vi "Config CDMA Trigger.vi"(0 "VISA Resource Name":refnum<visa-resource-name>, 1 "Delay State (F: OFF)":bool, 2 "External Delay (0.002)":dbl=0.002, 5 "Trigger Source  (0: KEY)":u16(ring) items=["KEY", "External", "BUS"], 7 "Trigger Type  (0: Continuous)":i16(ring) items=["Continuous", "Single", "Gate", "Segment Advance"], 9 "Gate Active  (0: Low)":i16(ring) items=["Low", "High"], 11 "error in (no error)":errorcluster {"code" format="%.0x"}, 12 "External Polarity  (1: Negative)":i16(ring)=1 items=["Positive", "Negative"]) -> (4 "VISA Resource Name Out":refnum<visa-resource-name>, 15 "error out":errorcluster {"code" format="%.0x"})   [LabVIEW 2014, in "Agilent ESG Series.lvlib"]
doc: "This VI configures CDMA trigger parameters.\n\nNotes:\n(1) This VI is supported for Agilent E44xxB with options UND and UN5 or E4438C with option 401 only."
uses:
  Agilent ESG Series.lvlib
panel:
  # "ON"
  # "OFF"
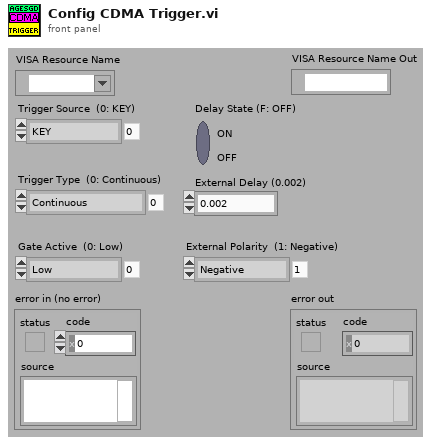
[diagram p1: front panel]
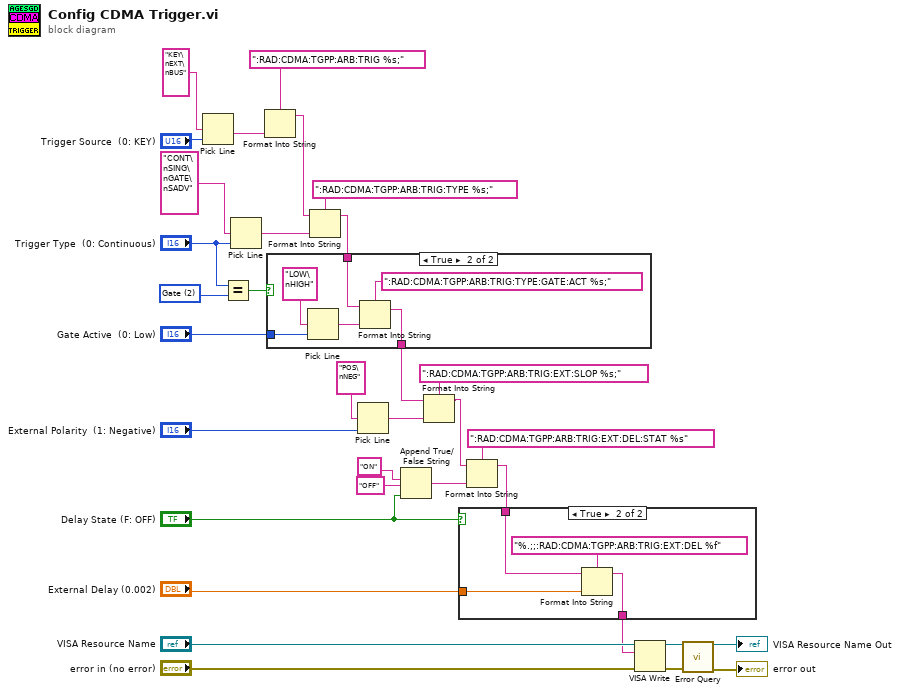
[diagram p0: block diagram]
diagram:
  w2 = i16 2 items=["Continuous", "Single", "Gate", "Segment Advance"] ("Trigger Type  (0: Continuous)")
  n1 = Pick Line(multi-line string="KEY\nEXT\nBUS", line index="Trigger Source  (0: KEY)") -> (output string=w10:string)  [unwired: 1 in]
  n2 = Equal?(x="Trigger Type  (0: Continuous)", y=w2) -> (x = y?=w3:bool)
  n3 = Pick Line(multi-line string="CONT\nSING\nGATE\nSADV", line index="Trigger Type  (0: Continuous)") -> (output string=w14:string)  [unwired: 1 in]
  n4 = Format Into String(format string=":RAD:CDMA:TGPP:ARB:TRIG %s;", w10) -> (resulting string=w4:string)  [unwired: 2 in, 1 out]
  n5 = Format Into String(format string=":RAD:CDMA:TGPP:ARB:TRIG:TYPE %s;", initial string=w4, w14) -> (resulting string=w5:string)  [unwired: 1 in, 1 out]
  n6 = case shown="True" w3 {
    tunnel: "Gate Active  (0: Low)" -> [_ w37]
    tunnel: [w34 w36] -> w6
    tunnel: w5 -> [w34 w35]
    frame False {
    }
    frame True {
      n7 = Pick Line(multi-line string="LOW\nHIGH", line index=w37) -> (output string=w38:string)  [unwired: 1 in]
      n8 = Format Into String(format string=":RAD:CDMA:TGPP:ARB:TRIG:TYPE:GATE:ACT %s;", initial string=w35, w38) -> (resulting string=w36:string)  [unwired: 1 in, 1 out]
    }
  }
  n9 = Pick Line(multi-line string="POS\nNEG", line index="External Polarity  (1: Negative)") -> (output string=w26:string)  [unwired: 1 in]
  n10 = Append True/False String(1:"Delay State (F: OFF)", 2:"OFF" ("false string"), 3:"ON" ("multi-line string")) -> (0:w20:string)  [unwired: 1 in]
  n11 = Format Into String(format string=":RAD:CDMA:TGPP:ARB:TRIG:EXT:SLOP %s;", initial string=w6, w26) -> (resulting string=w7:string)  [unwired: 1 in, 1 out]
  n12 = Format Into String(format string=":RAD:CDMA:TGPP:ARB:TRIG:EXT:DEL:STAT %s", initial string=w7, w20) -> (resulting string=w16:string)  [unwired: 1 in, 1 out]
  n13 = case shown="True" "Delay State (F: OFF)" {
    tunnel: "External Delay (0.002)" -> [_ w44]
    tunnel: w16 -> [w41 w43]
    tunnel: [w41 w42] -> w8
    frame False {
    }
    frame True {
      n14 = Format Into String(format string="%.;;:RAD:CDMA:TGPP:ARB:TRIG:EXT:DEL %f", initial string=w43, w44) -> (resulting string=w42:string)  [unwired: 1 in, 1 out]
    }
  }
  n15 = VISA Write(VISA resource name="VISA Resource Name", write buffer=w8, error in (no error)="error in (no error)") -> (VISA resource name out=w29:refnum<visa-resource-name>, error out=w28:errorcluster)  [unwired: 1 out]
  n16 = call "Error Query.vi"("VISA Resource Name"=w29, "error in (no error)"=w28) -> ("VISA Resource Name Out"=→"VISA Resource Name Out":refnum<visa-resource-name>, "error out"=→"error out":errorcluster)  [unwired: 10 in, 2 out]
